vi "Get Size.vi"(8 "error in (no error)":errorcluster, 11 "Glyph Destination in":refnum<class "Glyph Canvas.lvclass">) -> (0 "error out":errorcluster, 2 "Size":cluster{"Width":u16, "Height":u16}, 3 "Glyph Destination out":refnum<class "Glyph Canvas.lvclass">)   [LabVIEW 2020, in "Glyph Drawer.lvlib" / "Glyph Canvas.lvclass"]
uses:
  Glyph Canvas.lvclass
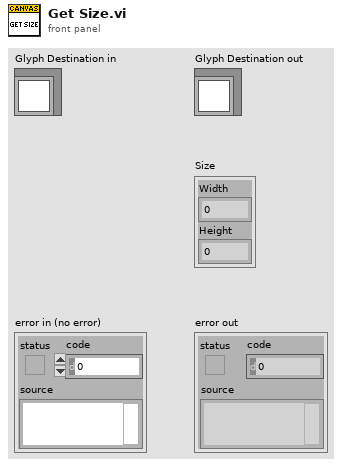
[diagram p1: front panel]
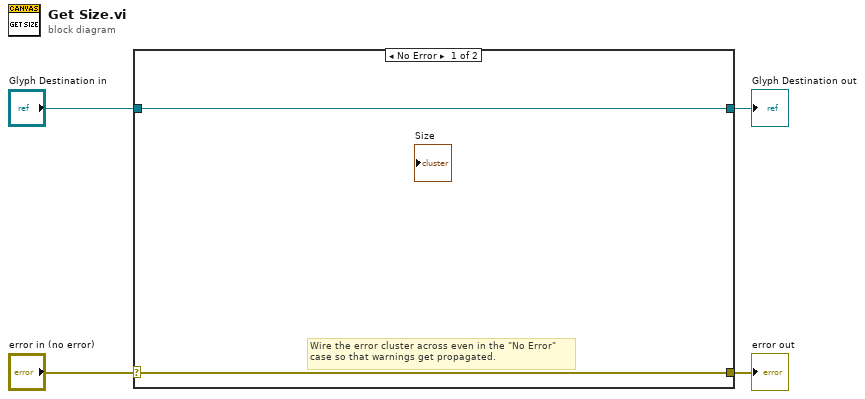
[diagram p0: block diagram]
diagram:
  n1 = case shown="No Error" "error in (no error)" {
    selector: "error in (no error)" -> [w5 w8]
    tunnel: [w5 w8] -> w3
    tunnel: [w6 w7] -> w1
    tunnel: "Glyph Destination in" -> [w6 w7]
    frame No Error {
      # "Wire the error cluster across even in the \"No Error\"\ncase so that warnings get propagated."
    }
    frame Error {
    }
  }
  "error out" <- w3
  "Glyph Destination out" <- w1
